vi "Bucket Summing.vi"(11 "Bucket Summing State In":enum16{"Reset", "Add To Bucket"}(ring)) -> (3 "Accumulation Complete?":bool)   [LabVIEW 2013]
doc: "Sums up the intensity for pixels within each sector."
uses:
  Globals/Accumulated Sector Intensity.vi
  <vilib>/rvi/Memory/Memory_Emulation/nirvimemoryFastEmulationFpgaImpl.vi
  <instcachedir>/0/nirvimemoryFastEmulationFpgaImpl_5FBAB50466BC4C939F684F8805638BFC.lvgen/nirvimemoryFastEmulationFpgaImpl_5FBAB50466BC4C939F684F8805638BFC_006.vi
  <vilib>/rvi/DataTransferAndStorage/Container/Common/niFpgaContainerGetUniqueNameForEmu.vi
  <vilib>/rvi/Memory/Memory_Emulation/nirvimemoryFastEmulation.vi
  <vilib>/rvi/Memory/Memory_Emulation/nirvimemoryEmulation.vi
  <vilib>/rvi/FIFO/Fifo_Resource/nirvififoEmulationReadFpgaImpl.vi
  <vilib>/rvi/DataTransferAndStorage/Container/XNode/niFpgaContainer.xnode
  <vilib>/rvi/FIFO/Fifo_Resource/nirvififoEmulationRead.vi
panel:
  out "End of Data?":bool[](array[boolean])
  out "Current FIFO Check":u8
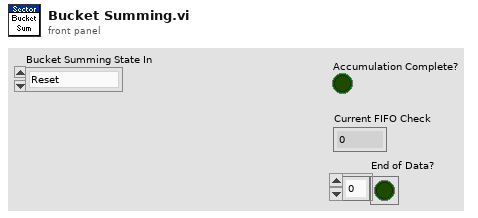
[diagram p1: front panel]
types:
  T1 = cluster{"Accumulated Intensity":u32, "Count":u16}
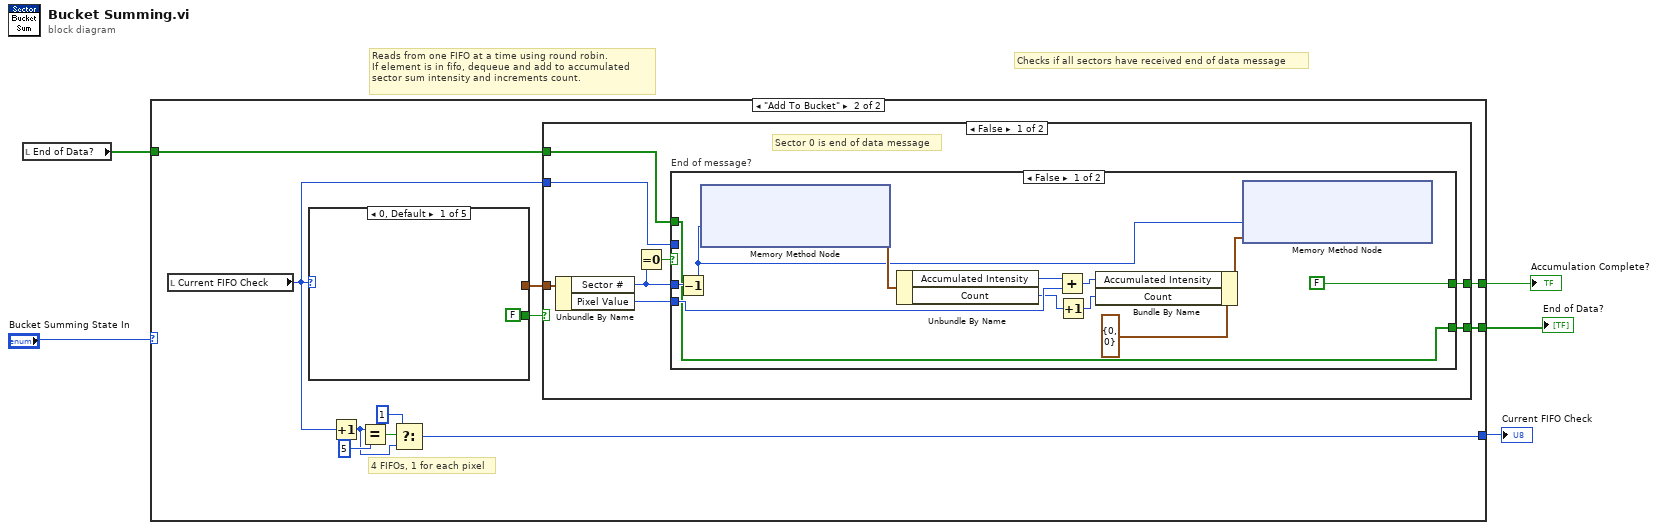
[diagram p0: block diagram]
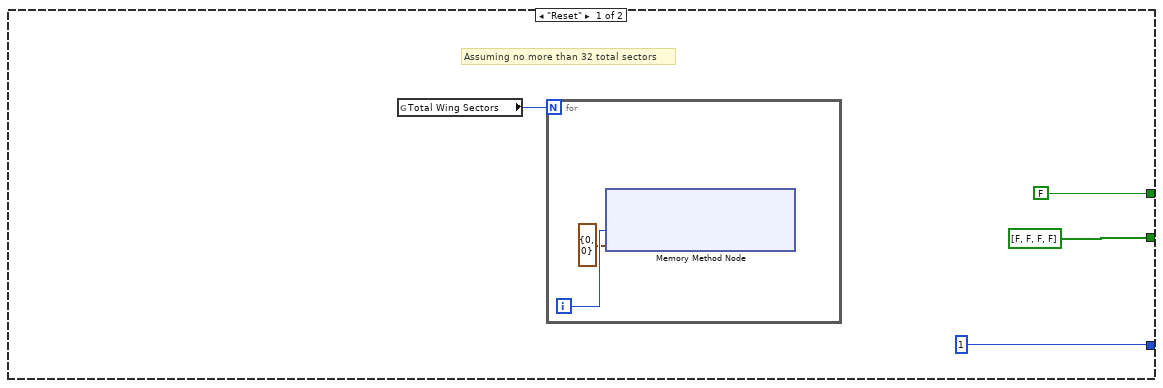
[diagram p2: hidden frame]
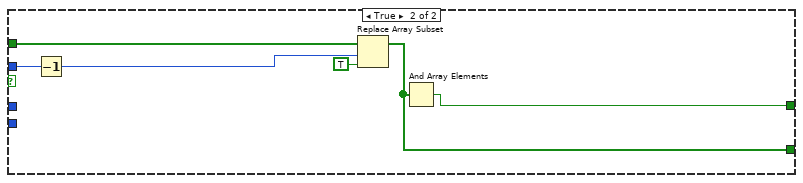
[diagram p3: hidden frame]
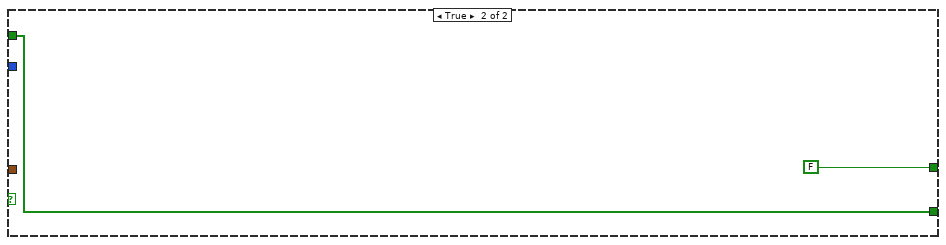
[diagram p4: hidden frame]
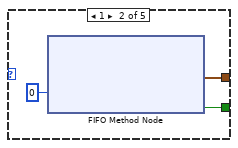
[diagram p5: hidden frame]
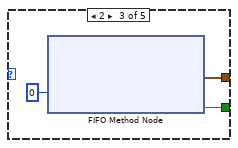
[diagram p6: hidden frame]
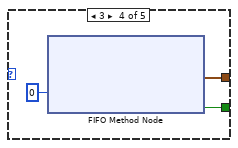
[diagram p7: hidden frame]
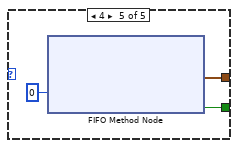
[diagram p8: hidden frame]
diagram:
  # "Checks if all sectors have received end of data message"
  # "Reads from one FIFO at a time using round robin.\nIf element is in fifo, dequeue and add to accumulated\nsector sum intensity and increments count."
  n1 = local read "End of Data?"() -> (w3:bool[])
  n2 = case shown="\"Add To Bucket\"" "Bucket Summing State In" {
    tunnel: [u8 1 ("Current FIFO Check") w16] -> w5
    tunnel: w3 -> [_ w14]
    tunnel: [FALSE w13] -> w2
    tunnel: [bool[] [FALSE, FALSE, FALSE, FALSE] ("End of Data?") w12] -> w1
    frame "Reset" {
      # "Assuming no more than 32 total sectors"
      n3 = global read "Accumulated Sector Intensity.vi" "Total Wing Sectors"() -> (w6:u8)
      n4 = for {
        N: w6 -> [_]
        i -> [w11]
        n5 = xnode ("Memory Method Node")("Address"=w11, "Data"=T1 {"Accumulated Intensity"=0, "Count"=0}) -> ()  [unwired: 1 in, 1 out]
      }
    }
    frame "Add To Bucket" {
      # "4 FIFOs, 1 for each pixel"
      n6 = local read "Current FIFO Check"() -> (w15:u8)
      n7 = case shown="0, Default" w15 {
        tunnel: [FALSE ("Timed Out?") w53 w56 w59 w62] -> w22
        tunnel: [_ w52 w55 w58 w61] -> w21
        frame 0, Default {
        }
        frame 1 {
          n8 = xnode ("FIFO Method Node")("Timeout"=0) -> ("Element"=w52:cluster{"Sector #":u8, "Pixel Value":u8}, "Timed Out?"=w53:bool)  [unwired: 1 in, 1 out]
        }
        frame 2 {
          n9 = xnode ("FIFO Method Node")("Timeout"=0) -> ("Element"=w55:cluster{"Sector #":u8, "Pixel Value":u8}, "Timed Out?"=w56:bool)  [unwired: 1 in, 1 out]
        }
        frame 3 {
          n10 = xnode ("FIFO Method Node")("Timeout"=0) -> ("Element"=w58:cluster{"Sector #":u8, "Pixel Value":u8}, "Timed Out?"=w59:bool)  [unwired: 1 in, 1 out]
        }
        frame 4 {
          n11 = xnode ("FIFO Method Node")("Timeout"=0) -> ("Element"=w61:cluster{"Sector #":u8, "Pixel Value":u8}, "Timed Out?"=w62:bool)  [unwired: 1 in, 1 out]
        }
      }
      n12 = Increment(x=w15) -> (x+1=w17:u8)
      n13 = Equal?(x=w17, y=u8 5) -> (x = y?=w19:bool)
      n14 = Select(t=u8 1 ("y"), s=w19, f=w17) -> (s? t:f=w16:u8)
      n15 = case shown="False" w22 {
        tunnel: w21 -> [w30 _]
        tunnel: w15 -> [w26 _]
        tunnel: w14 -> [w25 w49]
        tunnel: [w24 FALSE] -> w13
        tunnel: [w23 w49] -> w12
        frame False {
          # "Sector 0 is end of data message"
          n16 = Unbundle By Name(w30) -> ("Sector #"=w28:u8, "Pixel Value"=w29:u8)
          n17 = Equal To 0?(x=w28) -> (x = 0?=w27:bool)
          n18 = case "End of message?" shown="False" w27 {
            tunnel: w29 -> [w42 _]
            tunnel: w28 -> [w41 _]
            tunnel: w26 -> [_ w43]
            tunnel: w25 -> [w31 w48]
            tunnel: [FALSE w45] -> w24
            tunnel: [w31 w44] -> w23
            frame False {
              n19 = Decrement(x=w41) -> (x-1=w33:u8)
              n20 = xnode ("Memory Method Node")("Address"=w33) -> ("Data"=w34:T1)  [unwired: 1 in, 1 out]
              n21 = Unbundle By Name(w34) -> ("Accumulated Intensity"=w38:u32, "Count"=w35:u16)
              n22 = Add(x=w38, y=w42) -> (x+y=w37:u32)
              n23 = Increment(x=w35) -> (x+1=w36:u16)
              n24 = Bundle By Name(cluster=T1 {"Accumulated Intensity"=0, "Count"=0} ("element"), "Accumulated Intensity"=w37, "Count"=w36) -> (w32:T1)
              n25 = xnode ("Memory Method Node")("Address"=w33, "Data"=w32) -> ()  [unwired: 1 in, 1 out]
            }
            frame True {
              n26 = Decrement(x=w43) -> (x-1=w47:u8)
              n27 = Replace Array Subset(array=w48, new element=TRUE ("new element/subarray"), index=w47) -> (w44:bool[])
              n28 = And Array Elements(Boolean array=w44) -> (logical AND=w45:bool)
            }
          }
        }
        frame True {
        }
      }
    }
  }
  "Current FIFO Check" <- w5
  "Accumulation Complete?" <- w2
  "End of Data?" <- w1
